vi "tm3samp_02_sequence.vi"() -> ()   [LabVIEW 2023]
panel:
  out "DCAM Version":string
  out "Library Version":string
  out "Image":u16[][](graph)
  out "Frames Per Second":dbl
  in  "Quit":bool
  out "Error Out":errorcluster {"code" format="%.0x"}
  # "This is just a simple example\nof how to capture and display\nlive data."
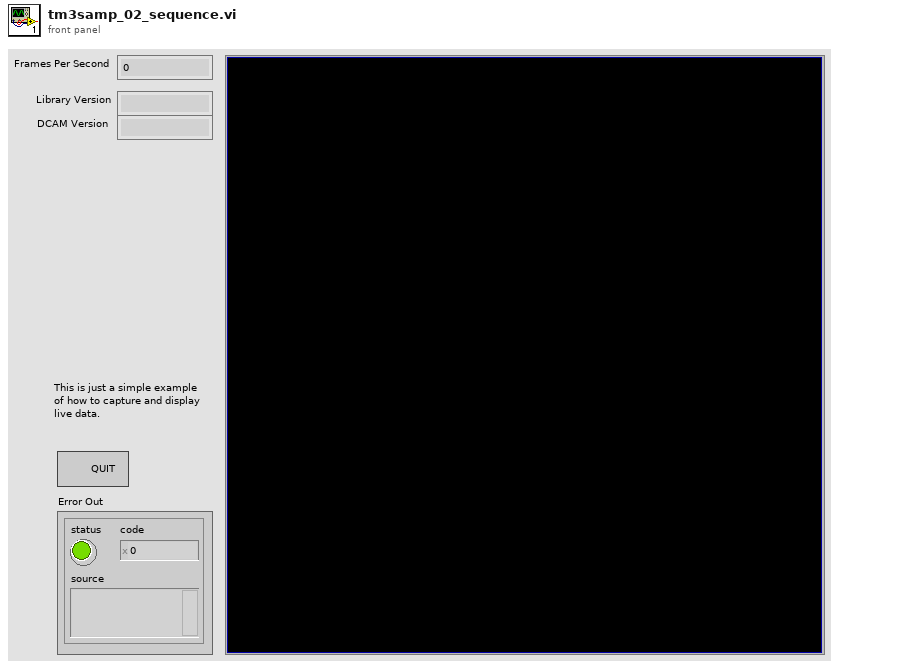
[diagram p1: front panel]
types:
  T1 = cluster{"Capture Library":string, "DCAM-API":string}
  T2 = cluster{"height":u32, "width":u32, "datatype":u32}
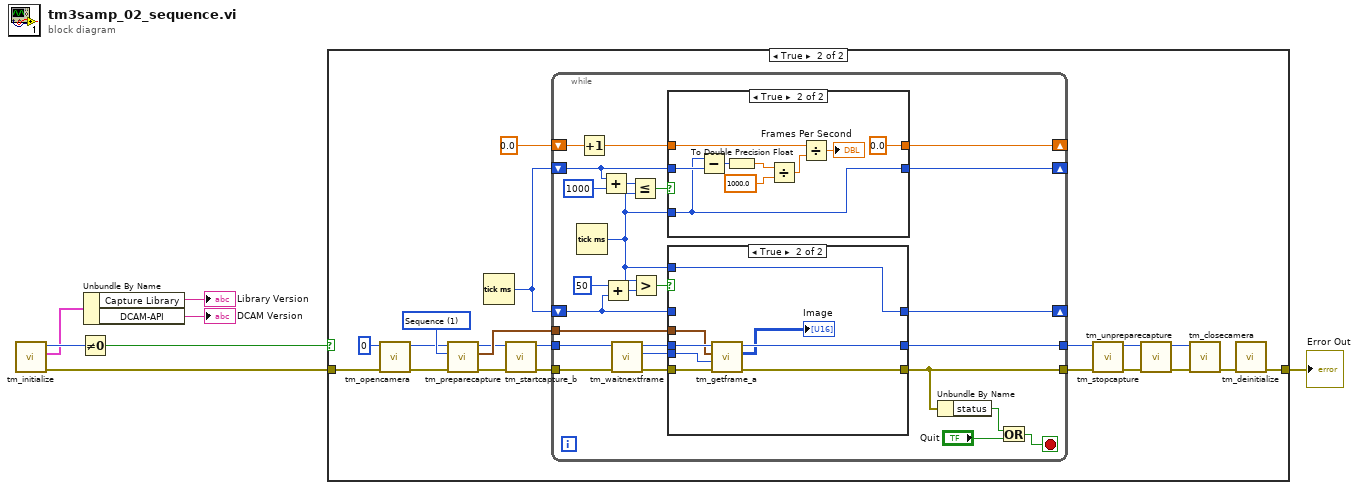
[diagram p0: block diagram]
diagram:
  n1 = call "tm_initialize.vi"() -> ("error out"=w4:errorcluster, "Version Info"=w3:T1, "Number Of Cameras"=w5:u32)  [unwired: 8 in, 1 out]
  n2 = Not Equal To 0?(x=w5) -> (x != 0?=w7:bool)
  n3 = Unbundle By Name(w3) -> ("Capture Library"=→"Library Version":string, "DCAM-API"=→"DCAM Version":string)
  n4 = case shown="True" w7 {
    tunnel: w4 -> [w8 w28]
    tunnel: [w8 w25] -> w6
    frame False {
    }
    frame True {
      w16 = 1 items=["Snap", "Sequence"] ("Capture mode")
      n5 = call "tm_opencamera.vi"("error in (no error)"=w28, "Camera Index"=u32 0) -> ("error out"=w9:errorcluster, "Handle out"=w10:u32)  [unwired: 7 in, 1 out]
      n6 = call "tm_preparecapture.vi"("error in (no error)"=w9, "Capture mode"=w16, "Handle in"=w10) -> ("error out"=w13:errorcluster, "Buffer Info"=w15:T2, "Handle out"=w14:u32)  [unwired: 5 in, 1 out]
      n7 = Tick Count (ms)() -> (millisecond timer value=w11:u32)
      n8 = call "tm_startcapture_b.vi"("error in (no error)"=w13, "Handle in"=w14) -> ("error out"=w17:errorcluster, "Handle out"=w18:u32)  [unwired: 8 in]
      n9 = while {
        tunnel: [w32] -> w21
        tunnel: [w33] -> w22
        tunnel: w15 -> [w30]
        tunnel: w18 -> [w50]
        tunnel: w17 -> [w51]
        shift-right: [w48] -> _
        shift-left: w11 -> [w45]
        shift-right: [w49] -> _
        shift-left: 0.0 -> [w42]
        shift-right: [w31] -> _
        shift-left: w11 -> [w34]
        stop <- w29 stop-if-true
        n10 = Tick Count (ms)() -> (millisecond timer value=w35:u32)
        n11 = Increment(x=w42) -> (x+1=w43:dbl)
        n12 = Add(x=w45, y=u32 1000) -> (x+y=w47:u32)
        n13 = Add(x=u32 50, y=w34) -> (x+y=w37:u32)
        n14 = call "tm_waitnextframe.vi"("error in (no error)"=w51, "Handle in"=w50) -> ("error out"=w40:errorcluster, "Frame Index"=w39:i32, "Handle out"=w41:u32)  [unwired: 6 in, 1 out]
        n15 = Less Or Equal?(x=w47, y=w35) -> (x <= y?=w44:bool)
        n16 = Greater?(x=w35, y=w37) -> (0:w36:bool)
        n17 = case shown="True" w44 {
          tunnel: w45 -> [w66 w69]
          tunnel: [w66 w67] -> w48
          tunnel: w43 -> [w65 w73]
          tunnel: w35 -> [_ w67]
          tunnel: [w65 0.0] -> w49
          frame False {
          }
          frame True {
            n18 = Subtract(x=w67, y=w69) -> (x-y=w68:u32)
            n19 = To Double Precision Float(number=w68) -> (double precision float=w75:dbl)
            n20 = Divide(x=w75, y=1000.0) -> (x/y=w72:dbl)
            n21 = Divide(x=w73, y=w72) -> (x/y=→"Frames Per Second":dbl)
          }
        }
        n22 = case shown="True" w36 {
          tunnel: w41 -> [w56 w64]
          tunnel: w40 -> [w55 w63]
          tunnel: w39 -> [_ w62]
          tunnel: w34 -> [w54 _]
          tunnel: w35 -> [_ w61]
          tunnel: [w56 w58] -> w32
          tunnel: [w55 w59] -> w33
          tunnel: [w54 w61] -> w31
          tunnel: w30 -> [_ w60]
          frame False {
          }
          frame True {
            n23 = call "tm_getframe_a.vi"("error in (no error)"=w63, "Frame Index"=w62, "Buffer Info"=w60, "Handle in"=w64) -> ("error out"=w59:errorcluster, "Data 16"=→"Image":u16[][], "Handle out"=w58:u32)  [unwired: 3 in, 2 out]
          }
        }
        n24 = Unbundle By Name(w33) -> ("status"=w53:bool)
        n25 = Or(x=w53, y="Quit") -> (x .or. y?=w29:bool)
      }
      n26 = call "tm_stopcapture.vi"("error in (no error)"=w22, "Handle in"=w21) -> ("error out"=w19:errorcluster, "Handle out"=w20:u32)  [unwired: 8 in]
      n27 = call "tm_unpreparecapture.vi"("error in (no error)"=w19, "Handle in"=w20) -> ("error out"=w24:errorcluster, "Handle out"=w23:u32)  [unwired: 8 in]
      n28 = call "tm_closecamera.vi"("error in (no error)"=w24, "Handle in"=w23) -> ("error out"=w26:errorcluster)  [unwired: 9 in]
      n29 = call "tm_deinitialize.vi"("error in (no error)"=w26) -> ("error out"=w25:errorcluster)  [unwired: 10 in]
    }
  }
  "Error Out" <- w6
